vi "ImportBehSession.vi"(8 "error in (no error)":errorcluster, 10 "Tuple":T1={"mouse_id"=1217.0, "session_timestamp"="", "trial_interval"=0.0, "response_interval"=0.0, "response_period"=0.0, "bad_delay"=0.0, "ExpType"="", "stimuli"="", "rewarded_stimuli"="", "setup"=0.0}, 11 "Database in":refnum<class "Database.lvclass">) -> (0 "error out":errorcluster, 3 "Database out":refnum<class "Database.lvclass">)   [LabVIEW 2014, in "Database.lvclass"]
uses:
  Database.lvclass
  Water Conditioning/ParamsTuple.ctl
  Database.lvclass/Database.ctl
  <vilib>/addons/database/NI_Database_API.lvlib
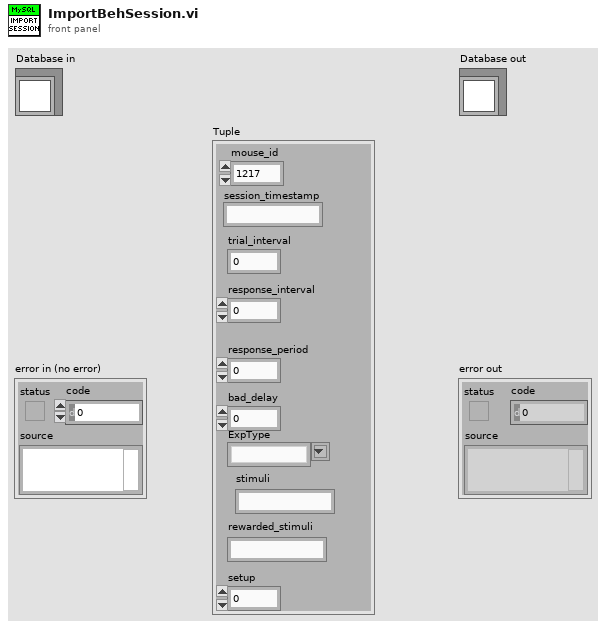
[diagram p1: front panel]
types:
  T1 = typedef "ParamsTuple.ctl" = cluster{"mouse_id":dbl, "session_timestamp":string, "trial_interval":dbl, "response_interval":dbl, "response_period":dbl, "bad_delay":dbl, "ExpType":string, "stimuli":string, "rewarded_stimuli":string, "setup":dbl}
  T2 = typedef "NI_Database_API.lvlib/Conn ObjectReference.ctl" = refnum<k1>
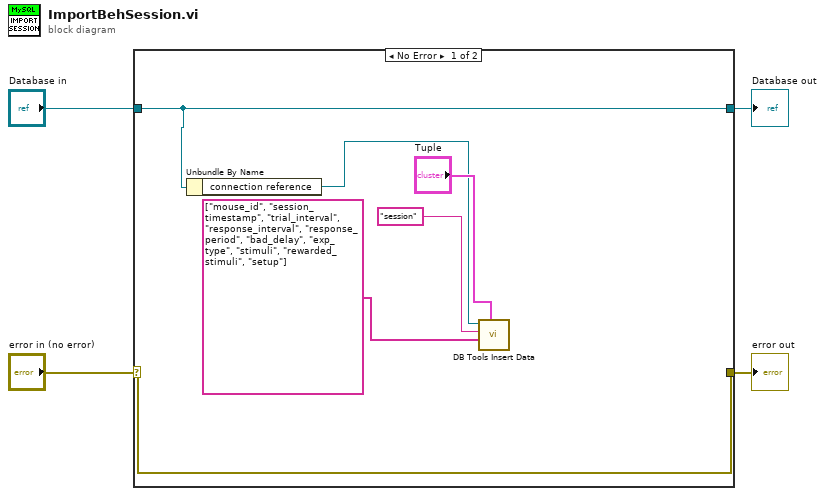
[diagram p0: block diagram]
diagram:
  n1 = case shown="No Error" "error in (no error)" {
    selector: "error in (no error)" -> [w10 w12]
    tunnel: [w10 w12] -> w3
    tunnel: [w6 w11] -> w1
    tunnel: "Database in" -> [w6 w11]
    frame No Error {
      n2 = Unbundle By Name(w6) -> ("connection reference"=w7:T2)
      n3 = call <vilib>:"DB Tools Insert Data.vi"("data"="Tuple", "columns"=string[] ["mouse_id", "session_timestamp", "trial_interval", "response_interval", "response_period", "bad_delay", "exp_type", "stimuli", "rewarded_stimuli", "setup"], "table"="session", "connection reference"=w7) -> ()  [unwired: 6 in, 2 out]
    }
    frame Error {
    }
  }
  "error out" <- w3
  "Database out" <- w1
